vi "Text control 2 v0.3.vi"() -> ()   [LabVIEW 2016]
panel:
  out "Ion vs time":cluster{"Y data in":dbl[], "X data in":dbl[]}[](graph)
  out "Ig":dbl format="%.2e"
  out "Id":dbl format="%.2e"
  out "Is":dbl format="%.2e"
  out "I vs Vg":cluster{"Y data in":dbl[], "X data in":dbl[]}[](graph)
  in  "Suffix":string=".txt"
  in  "Prefix":string="-transfer-"
  in  "Panel Controls 2":T1={"Emergency Stop"=refnum, "TransGraph Max"=1e-05, "Text/Graph (text=false)"=TRUE, "TransGraph Min"=1e-11} {"TransGraph Min" format="%.2e"; "TransGraph Max" format="%.2e"}
  out "Currently running:":string="#output s 0 0 0 -0.008 0.008 0.002"
  in  "Lines left to run:":string
  in  "Standby":T2
  in  "Full Reset":bool
  in  "SMU4":cluster{"on/off":bool, "Voltage":dbl} {"Voltage" min=-100.0 max=100.0 format="%.2f"}
  in  "Source/Drain\nRange":u8(slide)=6 max=11 scale=0.0..11.0
  in  "Source/Drain\nRange mode":u16(ring) items=["Auto", "Limited", "Fixed"]
  in  "Gate Range":u8(slide)=6 max=11 scale=0.0..11.0
  in  "Gate Range\nmode":u16(ring) items=["Auto", "Limited", "Fixed"]
  in  "Gate":T3={"Gate Start"=0.0, "Gate Stop"=2.0, "Gate Step (linear only)"=1.0, "Gate Compliance"=0.0001, "Gate PComp"=0.0, "Range mode"=0, "Range"=6} {"Range" max=11 scale=0.0..11.0; "Range mode" items=["Auto", "Limited", "Fixed"]; "Gate PComp" format="%^.2e"; "Gate Compliance" format="%^.2e"; "Gate Step (linear only)" format="%^.4e"; "Gate Stop" format="%^.4e"; "Gate Start" format="%^.4e"}
  in  "Drain 2":T4={"Drain Start"=0.0, "Drain Stop"=2.0, "Drain Compliance"=0.0001, "Drain Step"=1.0, "Drain PComp"=0.0, "Range mode"=0, "Range"=6} {"Range" max=11 scale=0.0..11.0; "Range mode" items=["Auto", "Limited", "Fixed"]; "Drain PComp" format="%^.2e"; "Drain Step" format="%^.4e"; "Drain Compliance" format="%^.2e"; "Drain Stop" format="%^.4e"; "Drain Start" format="%^.4e"}
  in  "Timings 2":T5={"integration time"=0, "Short/Long integration time"=0.00064, "hold time (sec)"=0.0, "delay time (sec)"=0.0, "Step Time (0 disables)"=0.0, "sweep method"=0, "Pulse period"=0.005, "Base voltage"=0.0, "Pulse width"=0.0005} {"Pulse width" min=0.0005 max=0.1 step=0.0001 format="%.4f"; "Base voltage" format="%^.4e"; "Pulse period" min=0.005 max=1.0 step=0.0001 format="%.4f"; "sweep method" items=["Continuous", "Pulsed"]; "Step Time (0 disables)" format="%.2f"; "delay time (sec)" format="%.4f"; "hold time (sec)" format="%.4f"; "Short/Long integration time" format="%^.0e"; "integration time" scale=0.0..2.0}
  in  "Panel Controls":T6={"Emergency Stop"=refnum, "TransGraph Max"=1e-05, "Text/Graph (text=false)"=TRUE} {"TransGraph Max" format="%.2e"}
  in  "Interrupt run":bool
  in  "Drain: Compliance":dbl=0.001 format="%.8f"
  in  "Gate: Compliance":dbl=0.001 format="%.8f"
  out "Path":path=path "C:/users/rlp38/09Apr2009LTtesting/test2.txt"
  in  "hold time /s":dbl format="%.2f"
  in  "delay time /s":dbl format="%.2f"
  in  "integration time":u32(slide) max=2 step=1 scale=0.0..2.0
  in  "Integration time (short)":dbl=0.0019 min=8e-05 max=0.0019 step=8e-05 format="%^.0e"
  in  "Integration time (long)":dbl=0.32 min=0.04 max=2.0 step=0.02 format="%.2f"
  in  "Step delay /s":dbl format="%.2f"
  in  "Program":string="#pulsedstressV d 0.03 20 0 0.5 0.0827 5\n#\n#itime m\n#gaterangemode a\n#drainrangemode a\n#pulsed on 0.05 0 0.02\n#transfer d -10 40 1 5 40 35\n#transfer d -10 40 1 5 40 35\n#transfer d -10 40 1 5 40 35\n#output d 0 40 20 0 40 1\n#\n#\n#sample 1 0.008 221 6 0.003\n#samplei 400e-6 200 6 0.002 0.1\n#vsu2pulse -10 4\n#\n#stressV 0.016 0.03 2e-4 0.1e-3 11\n#stressI 220e-7 0.08 15\n#transfer s -1 1 0.5 -0.005 0.005 0.005\n#output s 0 0 0 -0.008 0.008 0.002\n"
  # "Syntax:\nitime [s|m|l]\ngaterangemode [a|l|f]\ndrainrangemode [a|l|f]\npulsed [on|off] PulsePeriod(sec) PulseBaseVoltage PulseONWidth(sec)\nstandby [on l off]\nwait NumMilliseconds\nwait-min NumMinutes\n# texthere = comment\ntransfer [s|d] VgStart VgStop VgStep VdStart VdStop VdStep\noutput [s|d] VgStart VgStop VgStep VdStart VdStop VdStep\nsample Vg Vd NumSamples Time(s) SampleInterval(s)\nsamplei Idg NumSamples Time(s) SampleInterval(s) VDGcompliance\n# if in doubt use SampleInterval(s) = 0.004\nstressV VG VD IGcompliance IDcompliance Duration(sec)\nstressI IDG VDGcompliance Duration(sec)\nvsu2pulse Bias Duration(s)\npulsedstressV [s|d] VEstop VgON VgOFF Period(s) PulseONwidth(s) Vd\nsample-fpp Vg Vd NumSamples Time\nresample-fpp Vg Vd\ntransfer-fpp [s|d] VgStart VgStop VgStep VdStart VdStop VdStep\noutput-fpp [s|d] VgStart VgStop VgStep VdStart VdStop VdStep"
  # "100 samples is approx 13s with medium integration"
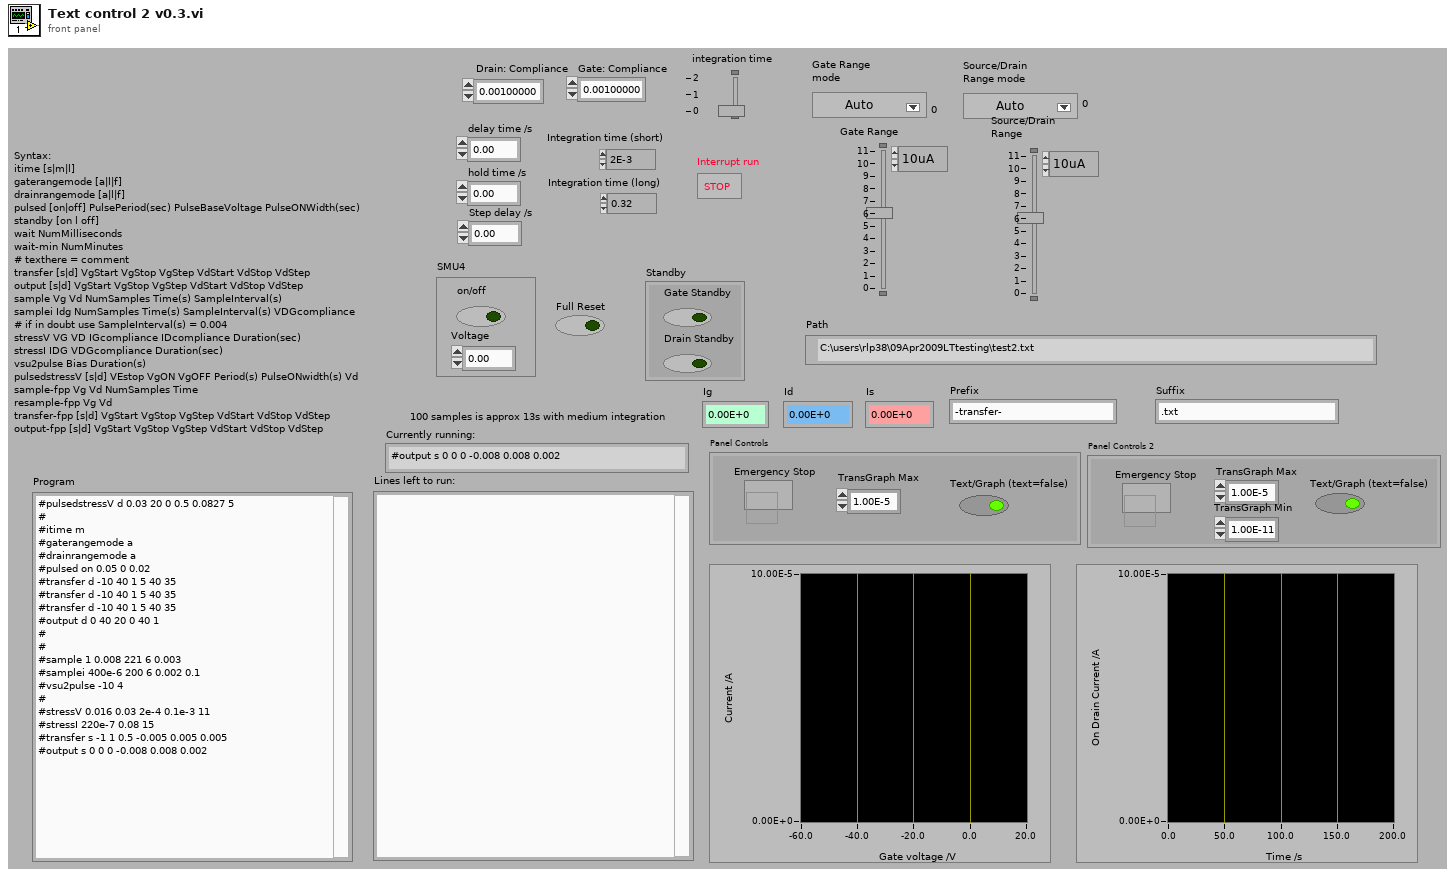
[diagram p1: front panel]
types:
  T1 = cluster{"Emergency Stop":refnum<vi>, "TransGraph Max":dbl, "Text/Graph (text=false)":bool, "TransGraph Min":dbl}
  T2 = cluster{"Gate Standby":bool, "Drain Standby":bool}
  T3 = cluster{"Gate Start":dbl, "Gate Stop":dbl, "Gate Step (linear only)":dbl, "Gate Compliance":dbl, "Gate PComp":dbl, "Range mode":u16, "Range":u8}
  T4 = cluster{"Drain Start":dbl, "Drain Stop":dbl, "Drain Compliance":dbl, "Drain Step":dbl, "Drain PComp":dbl, "Range mode":u16, "Range":u8}
  T5 = cluster{"integration time":u32, "Short/Long integration time":dbl, "hold time (sec)":dbl, "delay time (sec)":dbl, "Step Time (0 disables)":dbl, "sweep method":u16, "Pulse period":dbl, "Base voltage":dbl, "Pulse width":dbl}
  T6 = cluster{"Emergency Stop":refnum<vi>, "TransGraph Max":dbl, "Text/Graph (text=false)":bool}
  T7 = enum16{"open", "replace", "create", "open or create", "replace or create", "replace or create with confirmation"}
  T8 = cluster{"V2 Start":dbl, "V2 Step":dbl, "Number of points":i32}
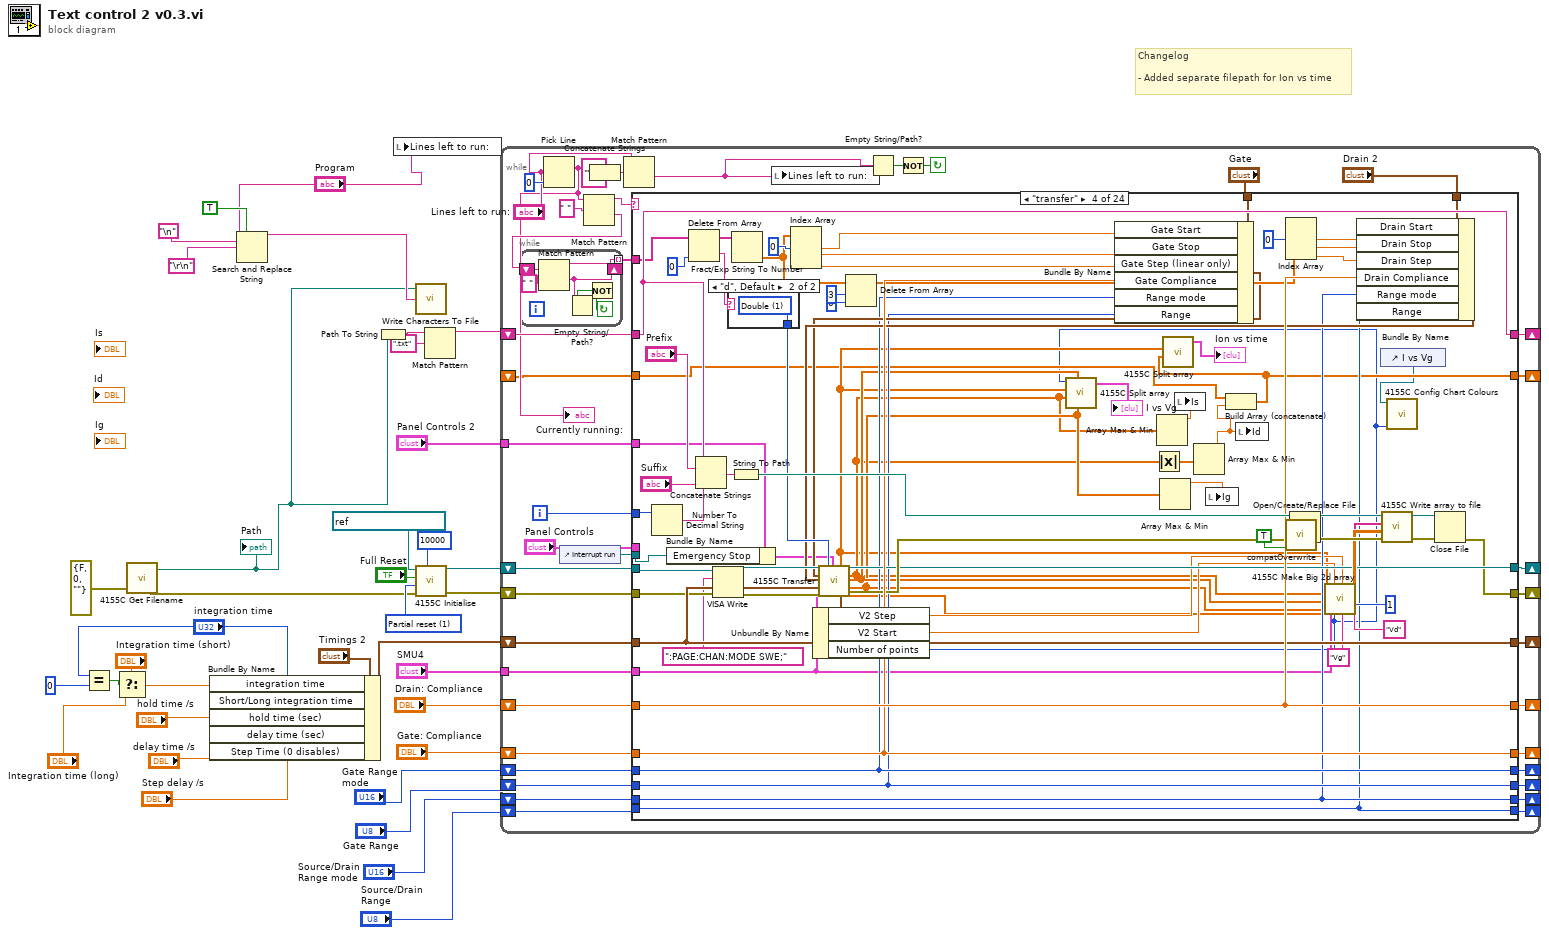
[diagram p0: block diagram]
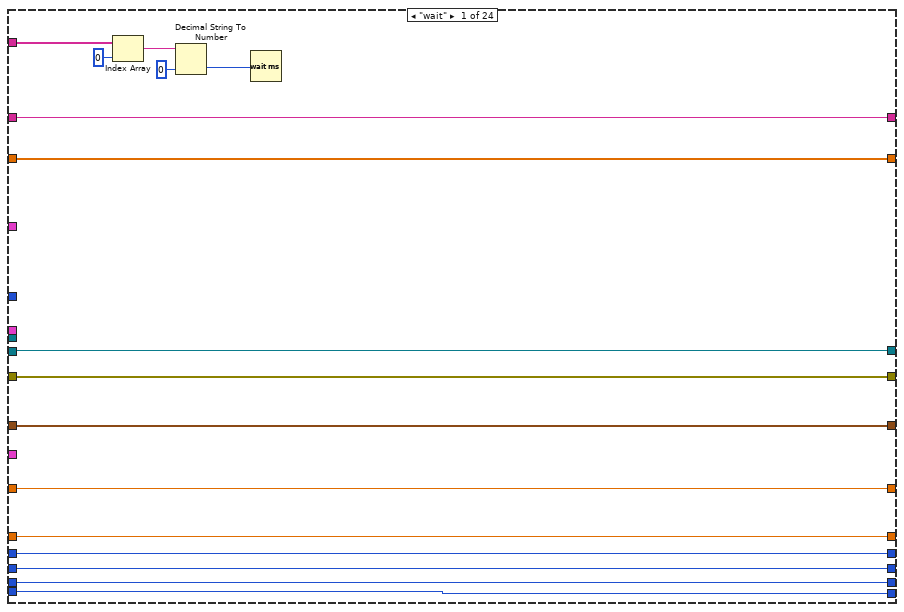
[diagram p2: hidden frame]
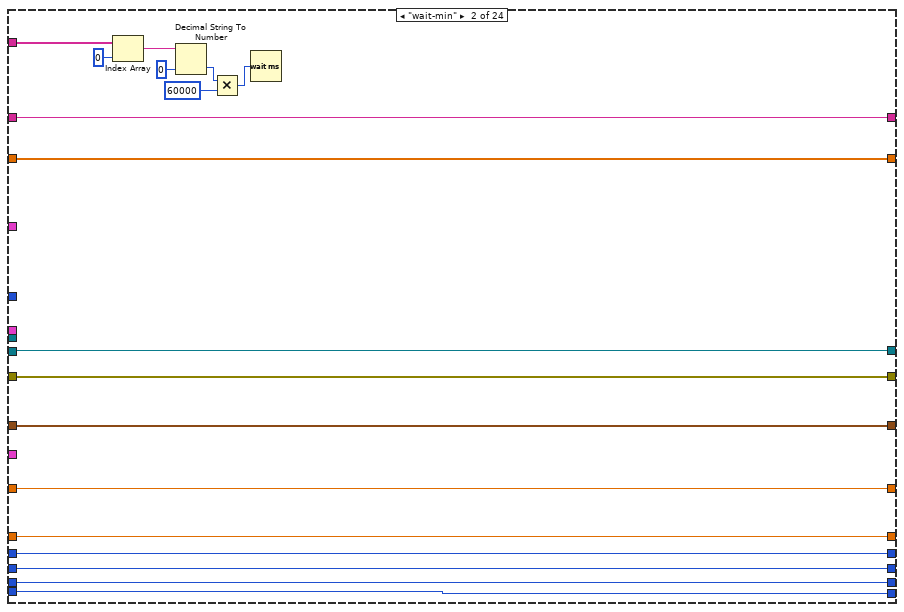
[diagram p3: hidden frame]
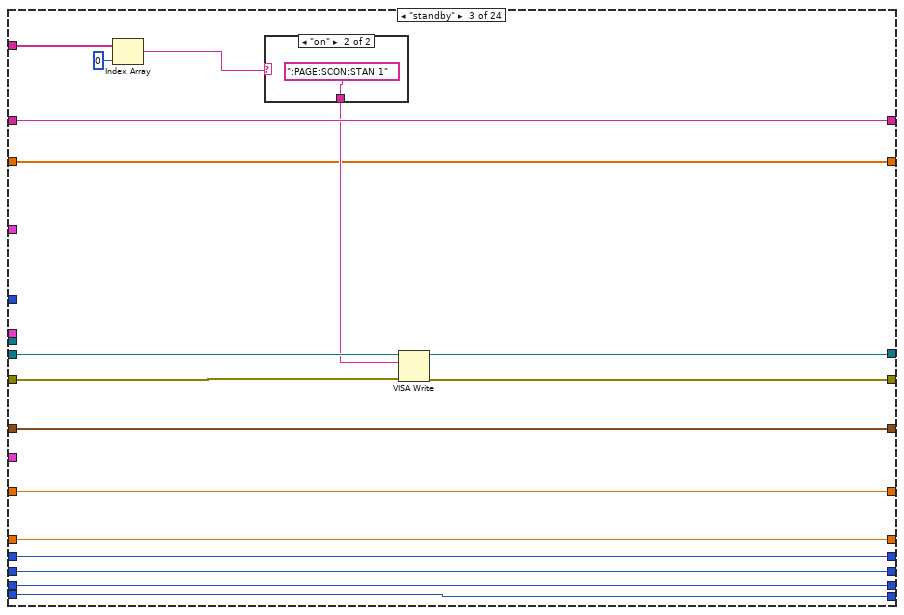
[diagram p4: hidden frame]
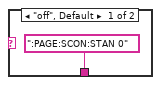
[diagram p5: hidden frame]
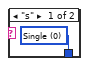
[diagram p6: hidden frame]
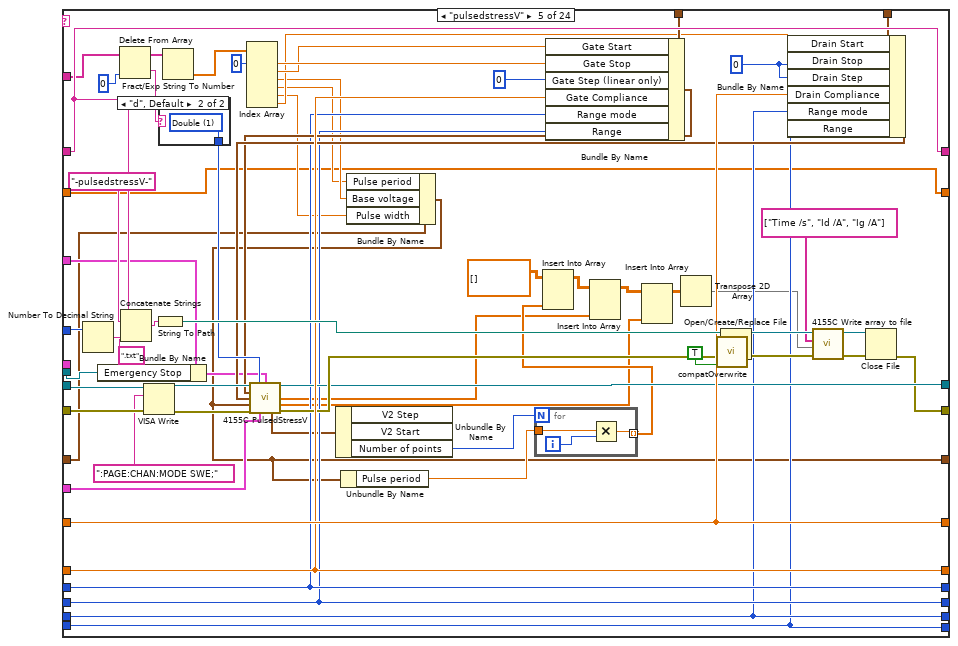
[diagram p7: hidden frame]
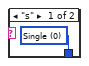
[diagram p8: hidden frame]
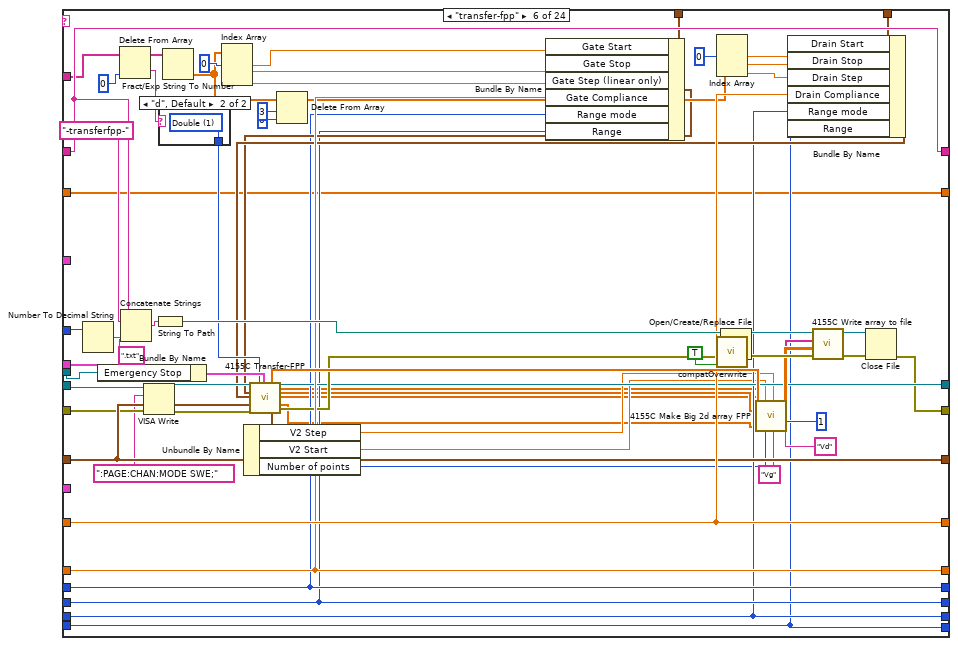
[diagram p9: hidden frame]
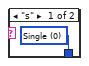
[diagram p10: hidden frame]
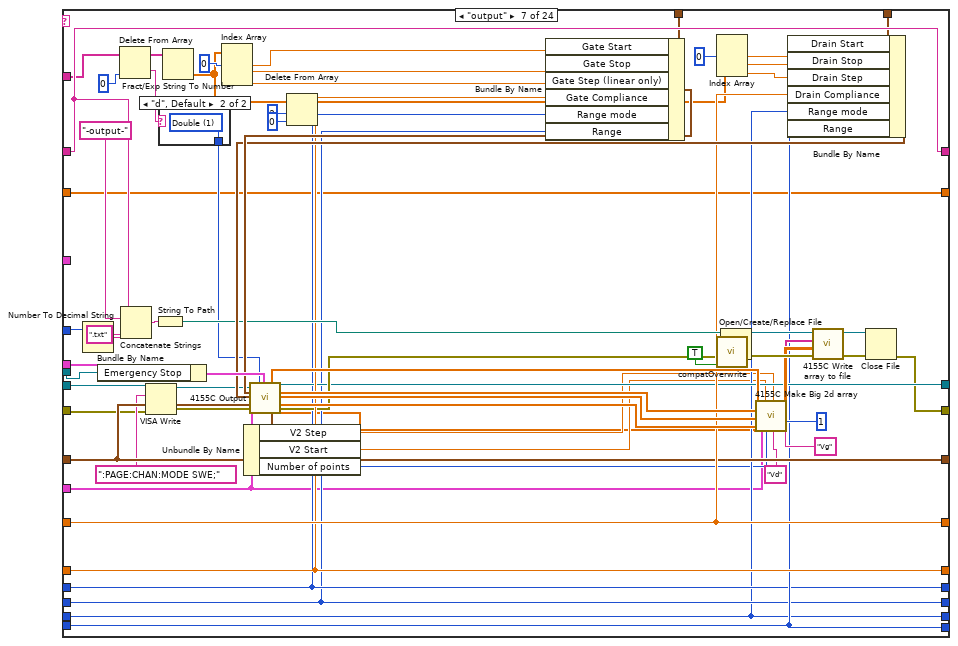
[diagram p11: hidden frame]
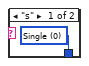
[diagram p12: hidden frame]
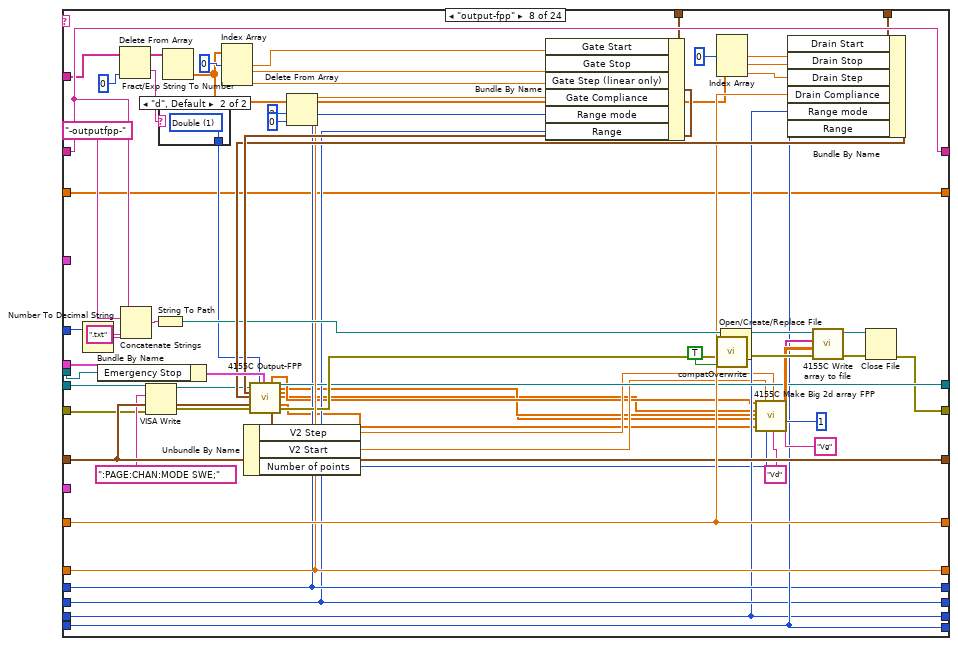
[diagram p13: hidden frame]
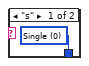
[diagram p14: hidden frame]
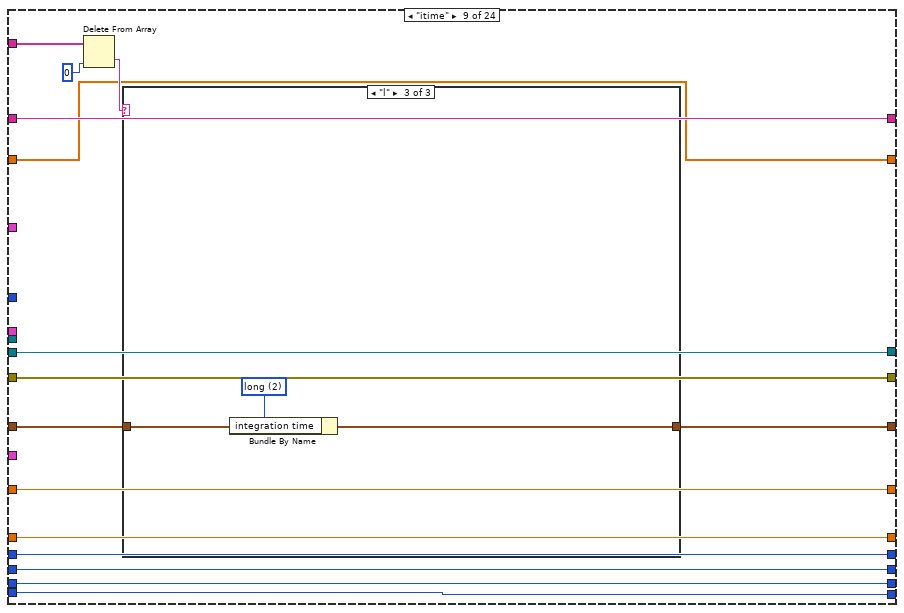
[diagram p15: hidden frame]
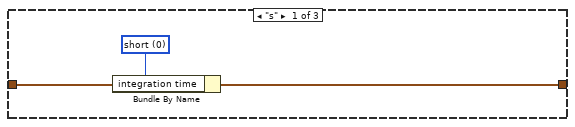
[diagram p16: hidden frame]
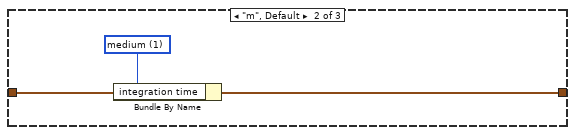
[diagram p17: hidden frame]
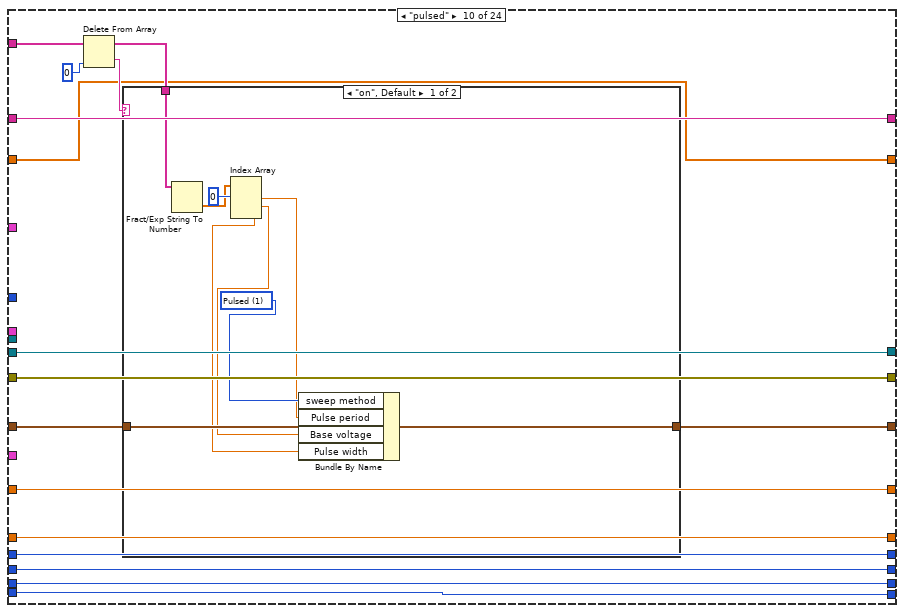
[diagram p18: hidden frame]
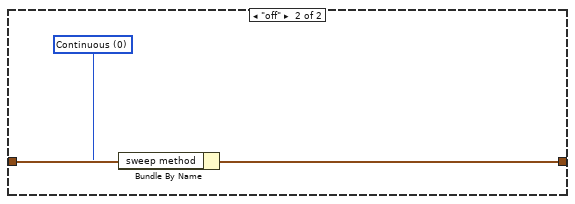
[diagram p19: hidden frame]
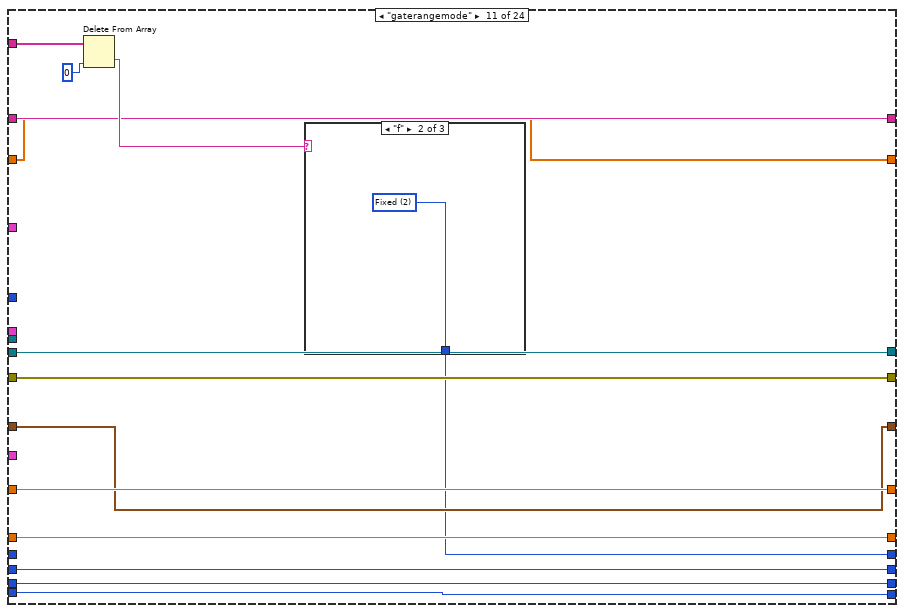
[diagram p20: hidden frame]
diagram:
  w27 = u16 1 items=["Reset All", "Partial reset"] ("Type of reset")
  # "Changelog\n\n- Added separate filepath for Ion vs time"
  n1 = Equal?(x="integration time", y=u32 0) -> (x = y?=w31:bool)
  n2 = Select(t="Integration time (short)", s=w31, f="Integration time (long)") -> (s? t:f=w35:dbl)
  n3 = call <userlib>:"4155C Get Filename.vi"("error in (no error)"=errorcluster {"status"=FALSE, "code"=0, "source"=""}) -> ("error out"=w22:errorcluster, "path"=w6:path)  [unwired: 2 in, 1 out]
  "Path" <- w6
  n4 = Bundle By Name(cluster="Timings 2", "integration time"="integration time", "Short/Long integration time"=w35, "hold time (sec)"="hold time /s", "delay time (sec)"="delay time /s", "Step Time (0 disables)"="Step delay /s") -> (w19:T5)
  n5 = Search and Replace String(replace all?=TRUE ("replace all? (F)"), input string="Program", search string="\n", replace string="\r\n") -> (result string=w9:string)  [unwired: 4 in, 3 out]
  n6 = Path To String(path=w6) -> (string=w5:string)
  n7 = local write "Lines left to run:"("Program") -> ()
  n8 = call <vilib>:"Write Characters To File.vi"("character string"=w9, "file path (dialog if empty)"=w6) -> ()  [unwired: 3 in, 1 out]
  n9 = call <userlib>:"4155C Initialise.vi"("VISA resource name in"=refnum<visa-resource-name> "GPIB0::14::INSTR", "Reset"="Full Reset", "Type of reset"=w27, "error in (no error)"=w22, "VISA Timeout Value"=u32 10000) -> ("VISA Resource Name out"=w21:refnum<visa-resource-name>, "error out"=w20:errorcluster)
  n10 = Match Pattern(string=w5, regular expression=".txt") -> (before substring=w4:string)  [unwired: 1 in, 3 out]
  n11 = while {
    tunnel: "SMU4" -> [w43]
    shift-left: "Source/Drain\nRange" -> [w48]
    shift-right: [w44] -> _
    shift-left: "Source/Drain\nRange mode" -> [w49]
    shift-right: [w45] -> _
    shift-left: "Gate Range" -> [w50]
    shift-right: [w46] -> _
    shift-left: "Gate Range\nmode" -> [w51]
    shift-right: [w47] -> _
    shift-left: "Gate: Compliance" -> [w63]
    shift-right: [w57] -> _
    shift-left: "Drain: Compliance" -> [w64]
    shift-right: [w58] -> _
    shift-left: w19 -> [w65]
    shift-right: [w59] -> _
    shift-left: w20 -> [w66]
    shift-right: [w60] -> _
    shift-left: w21 -> [w67]
    shift-right: [w61] -> _
    shift-left: w4 -> [w68]
    shift-right: [w56] -> _
    tunnel: "Panel Controls 2" -> [w39]
    shift-right: [w38] -> _
    shift-left: _ -> [w37]
    i -> [w62]
    stop <- w76 continue-if-true
    n12 = Pick Line(multi-line string="Lines left to run:", line index=0) -> (output string=w40:string)  [unwired: 1 in]
    "Currently running:" <- w40
    n13 = control-ref of="Interrupt run"() -> (w55:refnum<vi>)
    n14 = Match Pattern(string=w40, regular expression=" ") -> (before substring=w71:string, after substring=w70:string)  [unwired: 1 in, 2 out]
    n15 = while {
      tunnel: [w78] -> w69 mode=indexing
      shift-left: w70 -> [w80]
      shift-right: [w79] -> _
      stop <- w82 continue-if-true
      n16 = Match Pattern(string=w80, regular expression=" ") -> (before substring=w78:string, after substring=w79:string)  [unwired: 1 in, 2 out]
      n17 = Empty String/Path?(string/path=w79) -> (empty?=w83:bool)
      n18 = Not(x=w83) -> (.not. x?=w82:bool)
    }
    n19 = Concatenate Strings(w40, "\n" ("Substring")) -> (w74:string)
    n20 = Match Pattern(string="Lines left to run:", regular expression=w74) -> (after substring=w41:string)  [unwired: 1 in, 3 out]
    n21 = case shown="\"transfer\"" w71 {
      tunnel: w69 -> [w99 w117 w134 w193 w262 w329 w394 w467 w505 w530 w556 w580 w600 w613 _ _ w711 w770 _ w832 w874 w914 w982 w1042]
      tunnel: w68 -> [w94 w113 w132 w201 w269 w337 w402 w475 w494 w519 w548 w573 w594 w606 w624 w663 w689 w752 w783 w819 w861 w902 w976 w1038]
      tunnel: w67 -> [w93 w112 w123 w171 w253 w306 w370 w443 w495 w520 w549 w574 w595 w607 w629 w666 w718 w777 w787 w839 w881 w921 w989 w995]
      tunnel: w66 -> [w92 w111 w122 w170 w252 w305 w367 w440 w496 w521 w550 w575 w596 w608 w628 w635 w717 w776 w786 w838 w880 w920 w988 w994]
      tunnel: w65 -> [w91 w110 w131 w197 w227 w333 w398 w471 w504 w529 w547 w572 w593 w605 w627 w659 w680 w744 w792 w812 w854 w895 w975 w1037]
      tunnel: w64 -> [w90 w109 w130 w199 w267 w335 w400 w473 w503 w528 w555 w579 w599 w612 w626 w644 w716 w775 w795 w837 w879 w919 w987 w1047]
      tunnel: w63 -> [w89 w108 w129 w198 w266 w334 w399 w472 w502 w527 w554 w578 w598 w611 w625 w645 w690 w753 w794 w820 w862 w903 w977 w1039]
      tunnel: w62 -> [_ _ _ w139 w270 w338 w403 w476 _ _ _ _ _ _ _ w661 w715 w774 _ w836 w878 w918 w986 w1046]
      tunnel: [w93 w112 w121 w195 w264 w331 w396 w469 w495 w520 w549 w574 w595 w607 w629 w666 w681 w725 w785 w813 w855 w896 w927 w997] -> w61
      tunnel: [w92 w111 w120 w194 w263 w330 w395 w468 w496 w521 w550 w575 w596 w608 w628 w634 w691 w726 w784 w821 w863 w904 w926 w996] -> w60
      tunnel: [w91 w110 w131 w197 w223 w333 w398 w471 w497 w522 w547 w572 w593 w605 w627 w659 w680 w744 w792 w812 w854 w895 w975 w1037] -> w59
      tunnel: [w90 w109 w130 w199 w267 w335 w400 w473 w503 w528 w555 w579 w599 w612 w626 w644 w716 w775 w795 w837 w879 w919 w987 w1047] -> w58
      tunnel: [w89 w108 w129 w198 w266 w334 w399 w472 w502 w527 w554 w578 w598 w611 w625 w645 w690 w753 w794 w820 w862 w903 w977 w1039] -> w57
      tunnel: [w94 w113 w132 w201 w269 w337 w402 w475 w494 w519 w548 w573 w594 w606 w624 w663 w689 w752 w783 w819 w861 w902 w976 w1038] -> w56
      tunnel: w55 -> [_ _ _ w205 w274 w343 w411 w480 _ _ _ _ _ _ _ _ w686 w749 _ w818 w860 w901 w947 w1013]
      tunnel: "Gate" -> [_ _ _ w180 w256 w316 w381 w454 _ _ _ _ _ _ _ _ _ _ _ _ _ _ _ _]
      tunnel: "Drain 2" -> [_ _ _ w179 w255 w315 w380 w453 _ _ _ _ _ _ _ _ _ _ _ _ _ _ _ _]
      tunnel: "Panel Controls" -> [_ _ _ _ _ w314 w379 w452 _ _ _ _ _ _ _ _ _ _ _ _ _ _ _ _]
      tunnel: w51 -> [w88 w107 w128 w164 w246 w299 w365 w438 w501 w526 _ w571 w592 w604 w623 w646 w676 w740 w788 w808 w850 w891 w971 w1033]
      tunnel: w50 -> [w87 w106 w127 w163 w245 w298 w364 w437 w500 w525 w553 _ w583 w610 w622 w647 w677 w741 w789 w809 w851 w892 w972 w1034]
      tunnel: w49 -> [w86 w105 w126 w162 w244 w297 w363 w436 w499 w524 w552 w577 w597 _ w621 w648 w678 w742 w790 w810 w852 w893 w973 w1035]
      tunnel: w48 -> [w85 w104 w125 w161 w243 w296 w366 w439 w498 w523 w551 w576 _ w609 w620 w649 w679 w743 w791 w811 w853 w894 w974 w1036]
      tunnel: [w88 w107 w128 w164 w246 w299 w365 w438 w501 w526 w546 w571 w592 w604 w623 w646 w676 w740 w788 w808 w850 w891 w971 w1033] -> w47
      tunnel: [w87 w106 w127 w163 w245 w298 w364 w437 w500 w525 w553 w563 w583 w610 w622 w647 w677 w741 w789 w809 w851 w892 w972 w1034] -> w46
      tunnel: [w86 w105 w126 w162 w244 w297 w363 w436 w499 w524 w552 w577 w597 w603 w621 w648 w678 w742 w790 w810 w852 w893 w973 w1035] -> w45
      tunnel: [w85 w104 w125 w161 w243 w296 w366 w439 w498 w523 w551 w576 w584 w609 w620 w649 w679 w743 w791 w811 w853 w894 w974 w1036] -> w44
      tunnel: w43 -> [_ _ _ w155 w239 _ w357 _ _ _ _ _ _ _ _ _ _ _ _ _ _ _ _ _]
      tunnel: w39 -> [_ _ _ w153 w238 _ _ _ _ _ _ _ _ _ _ _ _ _ _ _ _ _ _ _]
      tunnel: [w84 w100 w118 w142 w215 w285 w354 w424 w493 w517 w545 w562 w582 w602 w619 w630 w667 w723 w782 w796 w842 w884 w924 w990] -> w38
      tunnel: w37 -> [w84 w100 w118 w141 w215 w285 w354 w424 w493 w517 w545 w562 w582 w602 w619 w630 w667 w723 w782 w796 w842 w884 w924 w990]
      frame "wait" {
        n22 = Index Array(array=w99, index=0 ("Index")) -> (element=w97:string)
        n23 = Decimal String To Number(string=w97, default (0L)=u32 0) -> (number=w96:u32)  [unwired: 1 in, 1 out]
        n24 = Wait (ms)(milliseconds to wait=w96) -> ()  [unwired: 1 out]
      }
      frame "wait-min" {
        n25 = Index Array(array=w117, index=0 ("Index")) -> (element=w115:string)
        n26 = Decimal String To Number(string=w115, default (0L)=u32 0) -> (number=w103:u32)  [unwired: 1 in, 1 out]
        n27 = Multiply(x=w103, y=u32 60000) -> (x*y=w102:u32)
        n28 = Wait (ms)(milliseconds to wait=w102) -> ()  [unwired: 1 out]
      }
      frame "standby" {
        n29 = Index Array(array=w134, index=0 ("Index")) -> (element=w124:string)
        n30 = case shown="\"on\"" w124 {
          tunnel: [":PAGE:SCON:STAN 0" ":PAGE:SCON:STAN 1"] -> w119
          frame "off", Default {
          }
          frame "on" {
          }
        }
        n31 = VISA Write(VISA resource name=w123, write buffer=w119, error in (no error)=w122) -> (VISA resource name out=w121:refnum<visa-resource-name>, error out=w120:errorcluster)  [unwired: 1 out]
      }
      frame "transfer" {
        n32 = Number To Decimal String(number=w139) -> (decimal integer string=w202:string)  [unwired: 1 in]
        n33 = Bundle By Name(cluster=w153, "Emergency Stop"=w205) -> (w154:T1)
        n34 = Delete From Array(array=w193, index=0 ("Index")) -> (deleted portion=w191:string, array with subset deleted=w190:string[])  [unwired: 1 in]
        n35 = Concatenate Strings(w201, "Prefix", w202, "Suffix") -> (w204:string)
        n36 = VISA Write(VISA resource name=w171, write buffer=":PAGE:CHAN:MODE SWE;" ("write buffer (\"\")"), error in (no error)=w170) -> (VISA resource name out=w168:refnum<visa-resource-name>, error out=w169:errorcluster)  [unwired: 1 out]
        n37 = case shown="\"d\", Default" w191 {
          tunnel: [w213 w214] -> w189
          frame "s" {
            w213 = u16 0 items=["Single", "Double"] ("sweep mode")
          }
          frame "d", Default {
            w214 = u16 1 items=["Single", "Double"] ("sweep mode")
          }
        }
        n38 = String To Path(string=w204) -> (path=w200:path)
        n39 = Fract/Exp String To Number(string=w190) -> (number=w175:dbl[])  [unwired: 3 in, 1 out]
        n40 = Index Array(array=w175, index #1=0 ("Index")) -> (element #1=w188:dbl, element #2=w187:dbl, element #3=w186:dbl)  [unwired: 2 in]
        n41 = Delete From Array(array=w175, length=3 ("Length"), index=0 ("Index")) -> (array with subset deleted=w173:dbl[])  [unwired: 1 out]
        n42 = Bundle By Name(cluster=w180, "Gate Start"=w188, "Gate Stop"=w187, "Gate Step (linear only)"=w186, "Gate Compliance"=w198, "Range mode"=w164, "Range"=w163) -> (w165:T3)
        n43 = Index Array(array=w173, index #1=0 ("Index")) -> (element #1=w183:dbl, element #2=w182:dbl, element #3=w181:dbl)  [unwired: 2 in]
        n44 = call <vilib>:"compatOverwrite.vi"("overwrite (F)"=TRUE) -> ("overwrite?"=w152:T7)
        n45 = Bundle By Name(cluster=w179, "Drain Start"=w183, "Drain Stop"=w182, "Drain Step"=w181, "Drain Compliance"=w199, "Range mode"=w162, "Range"=w161) -> (w166:T4)
        n46 = call <userlib>:"4155C Transfer.vi"("VISA resource name in"=w168, "Gate"=w165, "Drain"=w166, "Timings"=w197, "error in (no error)"=w169, "SMU4"=w155, "sweep mode"=w189, "Panel Controls"=w154) -> ("VG"=w143:dbl[], "Outparams"=w159:T8, "VISA Resource Name out"=w195:refnum<visa-resource-name>, "IS"=w145:dbl[], "ID"=w150:dbl[], "IG"=w146:dbl[], "error out"=w196:errorcluster, "SMU4"=w156:dbl[])  [unwired: 12 in]
        n47 = Unbundle By Name(w159) -> ("V2 Step"=w158:dbl, "V2 Start"=w157:dbl, "Number of points"=w138:i32)
        n48 = call <userlib>:"4155C Split array.vi"("Number of VAR2 steps"=w138, "Y2 data in"=w150, "X data in"=w143, "Y1 data in"=w145, "Y3 data in"=w146) -> ("Array of clusters"=→"I vs Vg":cluster{"Y data in":dbl[], "X data in":dbl[]}[])  [unwired: 2 in, 1 out]
        n49 = Absolute Value(x=w145) -> (abs(x)=w149:dbl[])
        n50 = Array Max & Min(array=w145) -> (max value=w147:dbl)  [unwired: 3 out]
        n51 = Array Max & Min(array=w146) -> (max value=w148:dbl)  [unwired: 3 out]
        n52 = local write "Is"(w147) -> ()
        n53 = Array Max & Min(array=w149) -> (max value=w140:dbl)  [unwired: 3 out]
        n54 = local write "Ig"(w148) -> ()
        n55 = Build Array (concatenate)(w141, w140) -> (w142:dbl[])
        n56 = call <userlib>:"4155C Split array.vi"("X data in"=w143, "Y1 data in"=w142) -> ("Array of clusters"=→"Ion vs time":cluster{"Y data in":dbl[], "X data in":dbl[]}[])  [unwired: 5 in, 1 out]
        n57 = local write "Id"(w140) -> ()
        n58 = Open/Create/Replace File(file path (use dialog)=w200, error in=w196, operation (0:open)=w152) -> (refnum out=w210:refnum<file>, error out=w211:errorcluster)  [unwired: 3 in, 1 out]
        n59 = call <userlib>:"4155C Make Big 2d array.vi"("1D Var1"=w143, "1d IS"=w145, "1d ID"=w150, "1d IG"=w146, "1d SMU4"=w156, "SMU4"=w155, "VAR2 START"=w157, "Number of VAR2 steps"=w138, "VAR2 STEP"=w158, "VAR1 Name"="Vg", "Decimal places in header"=i8 1, "VAR2 Name"="Vd") -> ("Header array"=w206:string[], "Data array"=w207:dbl[][])  [unwired: 14 in]
        n60 = control-ref of="I vs Vg"() -> (w137:refnum<vi>)
        n61 = call <userlib>:"4155C Write array to file.vi"("Byte Stream File Refnum"=w210, "Header"=w206, "Data Array"=w207, "error in (no error)"=w211) -> ("dup refnum"=w208:refnum<file>, "error out"=w209:errorcluster)  [unwired: 1 in]
        n62 = call <userlib>:"4155C Config Chart Colours.vi"("Numeric"=w138, "XY Graph 2"=w137) -> ()  [unwired: 6 in]
        n63 = Close File(refnum=w208, error in=w209) -> (error out=w194:errorcluster)  [unwired: 1 out]
      }
      frame "pulsedstressV" {
        w221 = 0
        n64 = Number To Decimal String(number=w270) -> (decimal integer string=w271:string)  [unwired: 1 in]
        n65 = Bundle By Name(cluster=w238, "Emergency Stop"=w274) -> (w240:T1)
        n66 = Delete From Array(array=w262, index=0 ("Index")) -> (deleted portion=w260:string, array with subset deleted=w259:string[])  [unwired: 1 in]
        n67 = Concatenate Strings(w269, "-pulsedstressV-" ("Substring"), w271, ".txt" ("Substring")) -> (w273:string)
        n68 = VISA Write(VISA resource name=w253, write buffer=":PAGE:CHAN:MODE SWE;" ("write buffer (\"\")"), error in (no error)=w252) -> (VISA resource name out=w250:refnum<visa-resource-name>, error out=w251:errorcluster)  [unwired: 1 out]
        n69 = String To Path(string=w273) -> (path=w268:path)
        n70 = case shown="\"d\", Default" w260 {
          tunnel: [w283 w284] -> w258
          frame "s" {
            w283 = u16 0 items=["Single", "Double"] ("sweep mode")
          }
          frame "d", Default {
            w284 = u16 1 items=["Single", "Double"] ("sweep mode")
          }
        }
        n71 = Fract/Exp String To Number(string=w259) -> (number=w254:dbl[])  [unwired: 3 in, 1 out]
        n72 = Index Array(array=w254, index #1=0 ("Index")) -> (element #1=w230:dbl, element #2=w229:dbl, element #3=w226:dbl, element #4=w225:dbl, element #5=w224:dbl, element #6=w228:dbl)  [unwired: 5 in]
        n73 = Bundle By Name(cluster=w227, "Pulse period"=w225, "Base voltage"=w226, "Pulse width"=w224) -> (w223:T5)
        n74 = Unbundle By Name(w223) -> ("Pulse period"=w231:dbl)
        n75 = Bundle By Name(cluster=w256, "Gate Start"=w229, "Gate Stop"=w230, "Gate Step (linear only)"=0, "Gate Compliance"=w266, "Range mode"=w246, "Range"=w245) -> (w247:T3)
        n76 = call <vilib>:"compatOverwrite.vi"("overwrite (F)"=TRUE) -> ("overwrite?"=w216:T7)
        n77 = Bundle By Name(cluster=w255, "Drain Start"=w228, "Drain Stop"=w221, "Drain Step"=w221, "Drain Compliance"=w267, "Range mode"=w244, "Range"=w243) -> (w248:T4)
        n78 = call <userlib>:"4155C PulsedStressV.vi"("VISA resource name in"=w250, "sweep mode"=w258, "Panel Controls"=w240, "Gate"=w247, "Drain"=w248, "Timings"=w223, "error in (no error)"=w251, "SMU4"=w239) -> ("VISA Resource Name out"=w264:refnum<visa-resource-name>, "ID"=w219:dbl[], "IG"=w217:dbl[], "Outparams"=w241:T8, "error out"=w265:errorcluster)  [unwired: 3 in]
        n79 = Unbundle By Name(w241) -> ("Number of points"=w218:i32)  [unwired: 2 out]
        n80 = for {
          N: w218 -> [_]
          tunnel: [w280] -> w220 mode=indexing
          tunnel: w231 -> [w282]
          i -> [w281]
          n81 = Multiply(x=w282, y=w281) -> (x*y=w280:dbl)
        }
        n82 = Insert Into Array(array=dbl[][] [] ("Input Array"), new element=w220) -> (w232:dbl[][])  [unwired: 2 in]
        n83 = Insert Into Array(array=w232, new element=w219) -> (w237:dbl[][])  [unwired: 2 in]
        n84 = Insert Into Array(array=w237, new element=w217) -> (w236:dbl[][])  [unwired: 2 in]
        n85 = Transpose 2D Array(2D array=w236) -> (transposed array=w235:dbl[][])
        n86 = Open/Create/Replace File(file path (use dialog)=w268, error in=w265, operation (0:open)=w216) -> (refnum out=w277:refnum<file>, error out=w278:errorcluster)  [unwired: 3 in, 1 out]
        n87 = call <userlib>:"4155C Write array to file.vi"("Byte Stream File Refnum"=w277, "Header"=string[] ["Time /s", "Id /A", "Ig /A"], "Data Array"=w235, "error in (no error)"=w278) -> ("dup refnum"=w275:refnum<file>, "error out"=w276:errorcluster)  [unwired: 1 in]
        n88 = Close File(refnum=w275, error in=w276) -> (error out=w263:errorcluster)  [unwired: 1 out]
      }
      frame "transfer-fpp" {
        n89 = Number To Decimal String(number=w338) -> (decimal integer string=w339:string)  [unwired: 1 in]
        n90 = Bundle By Name(cluster=w314, "Emergency Stop"=w343) -> (w351:T6)
        n91 = Delete From Array(array=w329, index=0 ("Index")) -> (deleted portion=w327:string, array with subset deleted=w326:string[])  [unwired: 1 in]
        n92 = Concatenate Strings(w337, "-transferfpp-" ("Substring"), w339, ".txt" ("Substring")) -> (w341:string)
        n93 = VISA Write(VISA resource name=w306, write buffer=":PAGE:CHAN:MODE SWE;" ("write buffer (\"\")"), error in (no error)=w305) -> (VISA resource name out=w303:refnum<visa-resource-name>, error out=w304:errorcluster)  [unwired: 1 out]
        n94 = String To Path(string=w341) -> (path=w336:path)
        n95 = case shown="\"d\", Default" w327 {
          tunnel: [w352 w353] -> w325
          frame "s" {
            w352 = u16 0 items=["Single", "Double"] ("sweep mode")
          }
          frame "d", Default {
            w353 = u16 1 items=["Single", "Double"] ("sweep mode")
          }
        }
        n96 = Fract/Exp String To Number(string=w326) -> (number=w310:dbl[])  [unwired: 3 in, 1 out]
        n97 = Index Array(array=w310, index #1=0 ("Index")) -> (element #1=w324:dbl, element #2=w323:dbl, element #3=w322:dbl)  [unwired: 2 in]
        n98 = Delete From Array(array=w310, length=3 ("Length"), index=0 ("Index")) -> (array with subset deleted=w308:dbl[])  [unwired: 1 out]
        n99 = Bundle By Name(cluster=w316, "Gate Start"=w324, "Gate Stop"=w323, "Gate Step (linear only)"=w322, "Gate Compliance"=w334, "Range mode"=w299, "Range"=w298) -> (w300:T3)
        n100 = Index Array(array=w308, index #1=0 ("Index")) -> (element #1=w319:dbl, element #2=w318:dbl, element #3=w317:dbl)  [unwired: 2 in]
        n101 = call <vilib>:"compatOverwrite.vi"("overwrite (F)"=TRUE) -> ("overwrite?"=w286:T7)
        n102 = Bundle By Name(cluster=w315, "Drain Start"=w319, "Drain Stop"=w318, "Drain Step"=w317, "Drain Compliance"=w335, "Range mode"=w297, "Range"=w296) -> (w301:T4)
        n103 = call <userlib>:"4155C Transfer-FPP.vi"("VISA resource name in"=w303, "Gate"=w300, "Drain"=w301, "Timings"=w333, "error in (no error)"=w304, "sweep mode"=w325, "Panel Controls"=w351) -> ("VG"=w342:dbl[], "Outparams"=w294:T8, "VISA Resource Name out"=w331:refnum<visa-resource-name>, "Vprobe2"=w290:dbl[], "ID"=w289:dbl[], "IG"=w288:dbl[], "Vprobe1"=w287:dbl[], "error out"=w332:errorcluster)  [unwired: 13 in]
        n104 = Unbundle By Name(w294) -> ("V2 Step"=w293:dbl, "V2 Start"=w292:dbl, "Number of points"=w291:i32)
        n105 = Open/Create/Replace File(file path (use dialog)=w336, error in=w332, operation (0:open)=w286) -> (refnum out=w348:refnum<file>, error out=w349:errorcluster)  [unwired: 3 in, 1 out]
        n106 = call <userlib>:"4155C Make Big 2d array FPP.vi"("1D Var1"=w342, "1d ID"=w289, "1d Vp2"=w290, "1d IG"=w288, "1d Vp1"=w287, "VAR2 START"=w292, "Number of VAR2 steps"=w291, "VAR2 STEP"=w293, "VAR1 Name"="Vg", "Decimal places in header"=i8 1, "VAR2 Name"="Vd") -> ("Header array"=w344:string[], "Data array"=w345:dbl[][])  [unwired: 15 in]
        n107 = call <userlib>:"4155C Write array to file.vi"("Byte Stream File Refnum"=w348, "Header"=w344, "Data Array"=w345, "error in (no error)"=w349) -> ("dup refnum"=w346:refnum<file>, "error out"=w347:errorcluster)  [unwired: 1 in]
        n108 = Close File(refnum=w346, error in=w347) -> (error out=w330:errorcluster)  [unwired: 1 out]
      }
      frame "output" {
        n109 = Number To Decimal String(number=w403) -> (decimal integer string=w404:string)  [unwired: 1 in]
        n110 = Bundle By Name(cluster=w379, "Emergency Stop"=w411) -> (w421:T6)
        n111 = Delete From Array(array=w394, index=0 ("Index")) -> (deleted portion=w392:string, array with subset deleted=w391:string[])  [unwired: 1 in]
        n112 = Concatenate Strings(w402, "-output-" ("Substring"), w404, ".txt" ("Substring")) -> (w406:string)
        n113 = VISA Write(VISA resource name=w370, write buffer=":PAGE:CHAN:MODE SWE;" ("write buffer (\"\")"), error in (no error)=w367) -> (VISA resource name out=w369:refnum<visa-resource-name>, error out=w368:errorcluster)  [unwired: 1 out]
        n114 = String To Path(string=w406) -> (path=w401:path)
        n115 = case shown="\"d\", Default" w392 {
          tunnel: [w422 w423] -> w390
          frame "s" {
            w422 = u16 0 items=["Single", "Double"] ("sweep mode")
          }
          frame "d", Default {
            w423 = u16 1 items=["Single", "Double"] ("sweep mode")
          }
        }
        n116 = Fract/Exp String To Number(string=w391) -> (number=w373:dbl[])  [unwired: 3 in, 1 out]
        n117 = Index Array(array=w373, index #1=0 ("Index")) -> (element #1=w389:dbl, element #2=w388:dbl, element #3=w387:dbl)  [unwired: 2 in]
        n118 = Delete From Array(array=w373, length=3 ("Length"), index=0 ("Index")) -> (array with subset deleted=w372:dbl[])  [unwired: 1 out]
        n119 = Bundle By Name(cluster=w381, "Gate Start"=w389, "Gate Stop"=w388, "Gate Step (linear only)"=w387, "Gate Compliance"=w399, "Range mode"=w365, "Range"=w364) -> (w420:T3)
        n120 = Index Array(array=w372, index #1=0 ("Index")) -> (element #1=w384:dbl, element #2=w383:dbl, element #3=w382:dbl)  [unwired: 2 in]
        n121 = call <vilib>:"compatOverwrite.vi"("overwrite (F)"=TRUE) -> ("overwrite?"=w355:T7)
        n122 = Bundle By Name(cluster=w380, "Drain Start"=w384, "Drain Stop"=w383, "Drain Step"=w382, "Drain Compliance"=w400, "Range mode"=w363, "Range"=w366) -> (w419:T4)
        n123 = call <userlib>:"4155C Output.vi"("VISA resource name in"=w369, "Gate"=w420, "Drain"=w419, "Timings"=w398, "error in (no error)"=w368, "SMU4"=w357, "sweep mode"=w390, "Panel controls"=w421) -> ("VD"=w407:dbl[], "Outparams"=w360:T8, "VISA Resource Name out"=w396:refnum<visa-resource-name>, "IS"=w410:dbl[], "ID"=w409:dbl[], "IG"=w408:dbl[], "error out"=w397:errorcluster, "SMU4"=w356:dbl[])  [unwired: 12 in]
        n124 = Unbundle By Name(w360) -> ("V2 Step"=w361:dbl, "V2 Start"=w359:dbl, "Number of points"=w358:i32)
        n125 = Open/Create/Replace File(file path (use dialog)=w401, error in=w397, operation (0:open)=w355) -> (refnum out=w416:refnum<file>, error out=w417:errorcluster)  [unwired: 3 in, 1 out]
        n126 = call <userlib>:"4155C Make Big 2d array.vi"("1D Var1"=w407, "1d IS"=w410, "1d ID"=w409, "1d IG"=w408, "1d SMU4"=w356, "SMU4"=w357, "VAR2 START"=w359, "Number of VAR2 steps"=w358, "VAR2 STEP"=w361, "VAR1 Name"="Vd", "Decimal places in header"=i8 1, "VAR2 Name"="Vg") -> ("Header array"=w412:string[], "Data array"=w413:dbl[][])  [unwired: 14 in]
        n127 = call <userlib>:"4155C Write array to file.vi"("Byte Stream File Refnum"=w416, "Header"=w412, "Data Array"=w413, "error in (no error)"=w417) -> ("dup refnum"=w414:refnum<file>, "error out"=w415:errorcluster)  [unwired: 1 in]
        n128 = Close File(refnum=w414, error in=w415) -> (error out=w395:errorcluster)  [unwired: 1 out]
      }
      frame "output-fpp" {
        n129 = Number To Decimal String(number=w476) -> (decimal integer string=w477:string)  [unwired: 1 in]
        n130 = Bundle By Name(cluster=w452, "Emergency Stop"=w480) -> (w490:T6)
        n131 = Delete From Array(array=w467, index=0 ("Index")) -> (deleted portion=w465:string, array with subset deleted=w464:string[])  [unwired: 1 in]
        n132 = Concatenate Strings(w475, "-outputfpp-" ("Substring"), w477, ".txt" ("Substring")) -> (w479:string)
        n133 = VISA Write(VISA resource name=w443, write buffer=":PAGE:CHAN:MODE SWE;" ("write buffer (\"\")"), error in (no error)=w440) -> (VISA resource name out=w442:refnum<visa-resource-name>, error out=w441:errorcluster)  [unwired: 1 out]
        n134 = String To Path(string=w479) -> (path=w474:path)
        n135 = case shown="\"d\", Default" w465 {
          tunnel: [w491 w492] -> w463
          frame "s" {
            w491 = u16 0 items=["Single", "Double"] ("sweep mode")
          }
          frame "d", Default {
            w492 = u16 1 items=["Single", "Double"] ("sweep mode")
          }
        }
        n136 = Fract/Exp String To Number(string=w464) -> (number=w446:dbl[])  [unwired: 3 in, 1 out]
        n137 = Index Array(array=w446, index #1=0 ("Index")) -> (element #1=w462:dbl, element #2=w461:dbl, element #3=w460:dbl)  [unwired: 2 in]
        n138 = Delete From Array(array=w446, length=3 ("Length"), index=0 ("Index")) -> (array with subset deleted=w445:dbl[])  [unwired: 1 out]
        n139 = Bundle By Name(cluster=w454, "Gate Start"=w462, "Gate Stop"=w461, "Gate Step (linear only)"=w460, "Gate Compliance"=w472, "Range mode"=w438, "Range"=w437) -> (w489:T3)
        n140 = Index Array(array=w445, index #1=0 ("Index")) -> (element #1=w457:dbl, element #2=w456:dbl, element #3=w455:dbl)  [unwired: 2 in]
        n141 = call <vilib>:"compatOverwrite.vi"("overwrite (F)"=TRUE) -> ("overwrite?"=w425:T7)
        n142 = Bundle By Name(cluster=w453, "Drain Start"=w457, "Drain Stop"=w456, "Drain Step"=w455, "Drain Compliance"=w473, "Range mode"=w436, "Range"=w439) -> (w488:T4)
        n143 = call <userlib>:"4155C Output-FPP.vi"("VISA resource name in"=w442, "Gate"=w489, "Drain"=w488, "Timings"=w471, "error in (no error)"=w441, "sweep mode"=w463, "Panel controls"=w490) -> ("VD"=w430:dbl[], "Outparams"=w433:T8, "VISA Resource Name out"=w469:refnum<visa-resource-name>, "Vprobe2"=w429:dbl[], "ID"=w428:dbl[], "IG"=w427:dbl[], "Vprobe1"=w426:dbl[], "error out"=w470:errorcluster)  [unwired: 13 in]
        n144 = Unbundle By Name(w433) -> ("V2 Step"=w434:dbl, "V2 Start"=w432:dbl, "Number of points"=w431:i32)
        n145 = Open/Create/Replace File(file path (use dialog)=w474, error in=w470, operation (0:open)=w425) -> (refnum out=w485:refnum<file>, error out=w486:errorcluster)  [unwired: 3 in, 1 out]
        n146 = call <userlib>:"4155C Make Big 2d array FPP.vi"("1D Var1"=w430, "1d ID"=w428, "1d Vp2"=w429, "1d IG"=w427, "1d Vp1"=w426, "VAR2 START"=w432, "Number of VAR2 steps"=w431, "VAR2 STEP"=w434, "VAR1 Name"="Vd", "Decimal places in header"=i8 1, "VAR2 Name"="Vg") -> ("Header array"=w481:string[], "Data array"=w482:dbl[][])  [unwired: 15 in]
        n147 = call <userlib>:"4155C Write array to file.vi"("Byte Stream File Refnum"=w485, "Header"=w481, "Data Array"=w482, "error in (no error)"=w486) -> ("dup refnum"=w483:refnum<file>, "error out"=w484:errorcluster)  [unwired: 1 in]
        n148 = Close File(refnum=w483, error in=w484) -> (error out=w468:errorcluster)  [unwired: 1 out]
      }
      frame "itime" {
        n149 = Delete From Array(array=w505, index=0 ("Index")) -> (deleted portion=w506:string)  [unwired: 1 in, 1 out]
        n150 = case shown="\"l\"" w506 {
          tunnel: w504 -> [w510 w512 w515]
          tunnel: [w509 w511 w514] -> w497
          frame "s" {
            w508 = u32 0 items=["short  ", "medium  ", "long  "] ("integration time 2")
            n151 = Bundle By Name(cluster=w510, "integration time"=w508) -> (w509:T5)
          }
          frame "m", Default {
            w513 = u32 1 items=["short  ", "medium  ", "long  "] ("integration time 2")
            n152 = Bundle By Name(cluster=w512, "integration time"=w513) -> (w511:T5)
          }
          frame "l" {
            w516 = u32 2 items=["short  ", "medium  ", "long  "] ("integration time 2")
            n153 = Bundle By Name(cluster=w515, "integration time"=w516) -> (w514:T5)
          }
        }
      }
      frame "pulsed" {
        n154 = Delete From Array(array=w530, index=0 ("Index")) -> (deleted portion=w531:string, array with subset deleted=w518:string[])  [unwired: 1 in]
        n155 = case shown="\"on\", Default" w531 {
          tunnel: w529 -> [w541 w544]
          tunnel: [w540 w543] -> w522
          tunnel: w518 -> [w538 _]
          frame "on", Default {
            w539 = u16 1 items=["Continuous", "Pulsed"] ("sweep method")
            n156 = Fract/Exp String To Number(string=w538) -> (number=w536:dbl[])  [unwired: 3 in, 1 out]
            n157 = Index Array(array=w536, index #1=0 ("Index")) -> (element #1=w535:dbl, element #2=w534:dbl, element #3=w533:dbl)  [unwired: 2 in]
            n158 = Bundle By Name(cluster=w541, "sweep method"=w539, "Pulse period"=w535, "Base voltage"=w534, "Pulse width"=w533) -> (w540:T5)
          }
          frame "off" {
            w542 = u16 0 items=["Continuous", "Pulsed"] ("sweep method")
            n159 = Bundle By Name(cluster=w544, "sweep method"=w542) -> (w543:T5)
          }
        }
      }
      frame "gaterangemode" {
        n160 = Delete From Array(array=w556, index=0 ("Index")) -> (deleted portion=w557:string)  [unwired: 1 in, 1 out]
        n161 = case shown="\"f\"" w557 {
          tunnel: [w559 w560 w561] -> w546
          frame "a", Default {
            w559 = u16 0 items=["Auto", "Limited", "Fixed"] ("Gate Range\nmode 2")
          }
          frame "f" {
            w560 = u16 2 items=["Auto", "Limited", "Fixed"] ("Gate Range\nmode 2")
          }
          frame "l" {
            w561 = u16 1 items=["Auto", "Limited", "Fixed"] ("Gate Range\nmode 2")
          }
        }
      }
      frame "gaterange" {
        (unwired) u8 11 items=["10fA  ", "100fA  ", "1nA  ", "10nA", "100nA", "1uA", "10uA", "100uA", "1mA", "10mA", "100mA", "1A"] ("Gate Range 2")
        n162 = Delete From Array(array=w580, index=0 ("Index")) -> (deleted portion=w570:string)  [unwired: 1 in, 1 out]
        n163 = Scan Value(string=w570, format string="") -> (value=w568:dbl)  [unwired: 1 in, 1 out]
        n164 = Logarithm Base 10(1:w568) -> (0:w567:dbl)
        n165 = Round To Nearest(number=w567) -> (nearest integer value=w566:dbl)
        n166 = Add(x=w566, y=11.0) -> (x+y=w564:dbl)
        n167 = To Unsigned Byte Integer(number=w564) -> (unsigned 8bit integer=w563:u8)
      }
      frame "drainrange" {
        (unwired) u8 11 items=["10fA  ", "100fA  ", "1nA  ", "10nA", "100nA", "1uA", "10uA", "100uA", "1mA", "10mA", "100mA", "1A"] ("Gate Range 2")
        n168 = Delete From Array(array=w600, index=0 ("Index")) -> (deleted portion=w591:string)  [unwired: 1 in, 1 out]
        n169 = Scan Value(string=w591, format string="") -> (value=w589:dbl)  [unwired: 1 in, 1 out]
        n170 = Logarithm Base 10(1:w589) -> (0:w588:dbl)
        n171 = Round To Nearest(number=w588) -> (nearest integer value=w587:dbl)
        n172 = Add(x=w587, y=11.0) -> (x+y=w585:dbl)
        n173 = To Unsigned Byte Integer(number=w585) -> (unsigned 8bit integer=w584:u8)
      }
      frame "drainrangemode" {
        n174 = Delete From Array(array=w613, index=0 ("Index")) -> (deleted portion=w614:string)  [unwired: 1 in, 1 out]
        n175 = case shown="\"f\"" w614 {
          tunnel: [w616 w617 w618] -> w603
          frame "a", Default {
            w616 = u16 0 items=["Auto", "Limited", "Fixed"] ("Gate Range\nmode 2")
          }
          frame "f" {
            w617 = u16 2 items=["Auto", "Limited", "Fixed"] ("Gate Range\nmode 2")
          }
          frame "l" {
            w618 = u16 1 items=["Auto", "Limited", "Fixed"] ("Gate Range\nmode 2")
          }
        }
      }
      frame "Error", Default {
      }
      frame "logfile" {
        n176 = Number To Decimal String(number=w661) -> (decimal integer string=w665:string)  [unwired: 1 in]
        n177 = Concatenate Strings(w663, "logfile" ("Substring"), w665, ".txt" ("Substring")) -> (w660:string)
        n178 = String To Path(string=w660) -> (path=w633:path)
        n179 = Unbundle(w659) -> ("integration time"=w658:u32, "Short/Long integration time"=w657:dbl, "hold time (sec)"=w656:dbl, "delay time (sec)"=w655:dbl, "Step Time (0 disables)"=w654:dbl, "sweep method"=w653:u16, "Pulse period"=w652:dbl, "Base voltage"=w651:dbl, "Pulse width"=w650:dbl)
        n180 = Build Array(w658, w657, w656, w655, w654, w653, w652, w651, w650, w644, w645, w646, w647, w648, w649) -> (w637:dbl[])
        n181 = Insert Into Array(array=dbl[][] [] ("Input Array"), new element=w637) -> (w636:dbl[][])  [unwired: 2 in]
        n182 = call <vilib>:"compatOverwrite.vi"("overwrite (F)"=TRUE) -> ("overwrite?"=w631:T7)
        n183 = Open/Create/Replace File(file path (use dialog)=w633, error in=w635, operation (0:open)=w631) -> (refnum out=w641:refnum<file>, error out=w640:errorcluster)  [unwired: 3 in, 1 out]
        n184 = call <userlib>:"4155C Write array to file.vi"("Byte Stream File Refnum"=w641, "Header"=string[] ["Int Time", "Short/Long Itime", "Hold time", "Delay time", "Step time", "Sweep method", "Pulse period", "Base Voltage", "Pulse width", "Drain compliance", "Gate compliance", "Gate range mode", "Gate range", "S/D range mode", "S/D range"], "Data Array"=w636, "error in (no error)"=w640) -> ("dup refnum"=w643:refnum<file>, "error out"=w642:errorcluster)  [unwired: 1 in]
        n185 = Close File(refnum=w643, error in=w642) -> (error out=w634:errorcluster)  [unwired: 1 out]
      }
      frame "sample" {
        n186 = Number To Decimal String(number=w715) -> (decimal integer string=w714:string)  [unwired: 1 in]
        n187 = Fract/Exp String To Number(string=w711) -> (number=w671:dbl[])  [unwired: 3 in, 1 out]
        n188 = Concatenate Strings(w689, "-sample-" ("Substring"), w714, ".txt" ("Substring")) -> (w712:string)
        n189 = String To Path(string=w712) -> (path=w693:path)
        n190 = Index Array(array=w671, index=0 ("Index")) -> (element=w709:dbl)
        n191 = Index Array(array=w671, index=2 ("Index")) -> (element=w705:dbl)
        n192 = Index Array(array=w671, index=3 ("Index")) -> (element=w674:dbl)
        n193 = Index Array(array=w671, index=4 ("Index")) -> (element=w670:dbl)
        n194 = call <userlib>:"4155C Config Sampling Measurements.vi"("Sampling interval"=w670, "Sample time"=w674, "Display on/off"=TRUE, "Timings"=w680, "Num Points"=w705, "error in (no error)"=w717, "Drain Compliance"=w716, "Gate Compliance"=w690, "VISA session"=w718) -> ("error out"=w719:errorcluster, "dup VISA resource name"=w720:refnum<visa-resource-name>)  [unwired: 1 in]
        n195 = Index Array(array=w671, index=1 ("Index")) -> (element=w706:dbl)
        n196 = call <userlib>:"4155C Take Sample.vi"("Emergency Stop"=w686, "error in (no error)"=w719, "Vd"=w706, "Vg"=w709, "VISA resource name in"=w720) -> ("error out"=w684:errorcluster, "Id"=w722:dbl[], "Ig"=w695:dbl[], "VISA Resource Name out"=w682:refnum<visa-resource-name>, "Is"=w721:dbl[], "Time"=w699:dbl[])  [unwired: 1 in]
        n197 = Insert Into Array(array=dbl[][] [] ("Input Array"), new element=w699) -> (w698:dbl[][])  [unwired: 2 in]
        n198 = Insert Into Array(array=w698, new element=w695) -> (w697:dbl[][])  [unwired: 2 in]
        n199 = Insert Into Array(array=w697, new element=w722) -> (w696:dbl[][])  [unwired: 2 in]
        n200 = VISA Write(VISA resource name=w682, write buffer=":DISP ON" ("write buffer (\"\")"), error in (no error)=w684) -> (VISA resource name out=w681:refnum<visa-resource-name>, error out=w683:errorcluster)  [unwired: 1 out]
        n201 = Insert Into Array(array=w696, new element=w721) -> (w688:dbl[][])  [unwired: 2 in]
        n202 = Transpose 2D Array(2D array=w688) -> (transposed array=w687:dbl[][])
        n203 = call <vilib>:"compatOverwrite.vi"("overwrite (F)"=TRUE) -> ("overwrite?"=w668:T7)
        n204 = Open/Create/Replace File(file path (use dialog)=w693, error in=w683, operation (0:open)=w668) -> (refnum out=w702:refnum<file>, error out=w701:errorcluster)  [unwired: 3 in, 1 out]
        n205 = call <userlib>:"4155C Write array to file.vi"("Byte Stream File Refnum"=w702, "Header"=string[] ["Time /s", "Ig /A", "Id /A", "Is /A"], "Data Array"=w687, "error in (no error)"=w701) -> ("dup refnum"=w704:refnum<file>, "error out"=w703:errorcluster)  [unwired: 1 in]
        n206 = Close File(refnum=w704, error in=w703) -> (error out=w691:errorcluster)  [unwired: 1 out]
      }
      frame "samplei" {
        n207 = Number To Decimal String(number=w774) -> (decimal integer string=w773:string)  [unwired: 1 in]
        n208 = Fract/Exp String To Number(string=w770) -> (number=w736:dbl[])  [unwired: 3 in, 1 out]
        n209 = Concatenate Strings(w752, "-samplei-" ("Substring"), w773, ".txt" ("Substring")) -> (w771:string)
        n210 = String To Path(string=w771) -> (path=w755:path)
        n211 = Index Array(array=w736, index=4 ("Index")) -> (element=w730:dbl)
        n212 = Index Array(array=w736, index=3 ("Index")) -> (element=w731:dbl)
        n213 = Index Array(array=w736, index=1 ("Index")) -> (element=w733:dbl)
        n214 = Index Array(array=w736, index=0 ("Index")) -> (element=w734:dbl)
        n215 = Index Array(array=w736, index=2 ("Index")) -> (element=w732:dbl)
        n216 = call <userlib>:"4155C Config SamplingI Measurements.vi"("Sample time"=w732, "Display on/off"=TRUE, "Timings"=w744, "Num Points"=w733, "error in (no error)"=w776, "Sampling interval"=w731, "VISA session"=w777) -> ("error out"=w778:errorcluster, "dup VISA resource name"=w779:refnum<visa-resource-name>)  [unwired: 3 in]
        n217 = call <userlib>:"4155C Take SampleI.vi"("Emergency Stop"=w749, "error in (no error)"=w778, "Idg 2"=w734, "Vdg compliance 2"=w730, "VISA resource name in"=w779) -> ("error out"=w747:errorcluster, "Idg"=w781:dbl[], "Vdg"=w757:dbl[], "VISA Resource Name out"=w745:refnum<visa-resource-name>, "Is"=w780:dbl[], "Time"=w761:dbl[])  [unwired: 1 in]
        n218 = Insert Into Array(array=dbl[][] [] ("Input Array"), new element=w761) -> (w760:dbl[][])  [unwired: 2 in]
        n219 = Insert Into Array(array=w760, new element=w757) -> (w759:dbl[][])  [unwired: 2 in]
        n220 = Insert Into Array(array=w759, new element=w781) -> (w758:dbl[][])  [unwired: 2 in]
        n221 = VISA Write(VISA resource name=w745, write buffer=":DISP ON" ("write buffer (\"\")"), error in (no error)=w747) -> (VISA resource name out=w729:refnum<visa-resource-name>, error out=w746:errorcluster)  [unwired: 1 out]
        n222 = Insert Into Array(array=w758, new element=w780) -> (w751:dbl[][])  [unwired: 2 in]
        n223 = Transpose 2D Array(2D array=w751) -> (transposed array=w750:dbl[][])
        n224 = call <vilib>:"compatOverwrite.vi"("overwrite (F)"=TRUE) -> ("overwrite?"=w724:T7)
        n225 = Open/Create/Replace File(file path (use dialog)=w755, error in=w746, operation (0:open)=w724) -> (refnum out=w764:refnum<file>, error out=w763:errorcluster)  [unwired: 3 in, 1 out]
        n226 = call <userlib>:"4155C Write array to file.vi"("Byte Stream File Refnum"=w764, "Header"=string[] ["Time /s", "Vdg /V", "Idg /A", "Is /A"], "Data Array"=w750, "error in (no error)"=w763) -> ("dup refnum"=w766:refnum<file>, "error out"=w765:errorcluster)  [unwired: 1 in]
        n227 = Close File(refnum=w766, error in=w765) -> (error out=w727:errorcluster)  [unwired: 1 out]
        n228 = VISA Write(VISA resource name=w729, write buffer=";:PAGE:SCON:STAN OFF;:PAGE:CHAN:VSU2:DIS;" ("write buffer (\"\")"), error in (no error)=w727) -> (VISA resource name out=w725:refnum<visa-resource-name>, error out=w726:errorcluster)  [unwired: 1 out]
      }
      frame "#" {
        n229 = VISA Write(VISA resource name=w787, write buffer=":DISP ON" ("write buffer (\"\")"), error in (no error)=w786) -> (VISA resource name out=w785:refnum<visa-resource-name>, error out=w784:errorcluster)  [unwired: 1 out]
      }
      frame "stressV" {
        n230 = Number To Decimal String(number=w836) -> (decimal integer string=w835:string)  [unwired: 1 in]
        n231 = Fract/Exp String To Number(string=w832) -> (number=w804:dbl[])  [unwired: 3 in, 1 out]
        n232 = Concatenate Strings(w819, "-stressV-" ("Substring"), w835, ".txt" ("Substring")) -> (w833:string)
        n233 = String To Path(string=w833) -> (path=w823:path)
        n234 = Index Array(array=w804, index=3 ("Index")) -> (element=w801:dbl)
        n235 = Index Array(array=w804, index=1 ("Index")) -> (element=w799:dbl)
        n236 = Index Array(array=w804, index=0 ("Index")) -> (element=w798:dbl)
        n237 = Index Array(array=w804, index=4 ("Index")) -> (element=w803:dbl)
        n238 = Index Array(array=w804, index=2 ("Index")) -> (element=w800:dbl)
        n239 = call <userlib>:"4155C Config V Stress.vi"("VISA session"=w839, "ID compliance"=w801, "VD"=w799, "VG"=w798, "IG compliance"=w800, "error in (no error)"=w838, "Display on/off"=TRUE) -> ("dup VISA resource name"=w841:refnum<visa-resource-name>, "error out"=w840:errorcluster)
        n240 = call <userlib>:"4155C Apply Stress.vi"("error in (no error)"=w840, "Duration"=w803, "Emergency Stop"=w818, "VISA resource name in"=w841) -> ("error out"=w816:errorcluster, "VISA Resource Name out"=w814:refnum<visa-resource-name>)
        n241 = VISA Write(VISA resource name=w814, write buffer=":DISP ON" ("write buffer (\"\")"), error in (no error)=w816) -> (VISA resource name out=w813:refnum<visa-resource-name>, error out=w815:errorcluster)  [unwired: 1 out]
        n242 = call <vilib>:"compatOverwrite.vi"("overwrite (F)"=TRUE) -> ("overwrite?"=w797:T7)
        n243 = Open/Create/Replace File(file path (use dialog)=w823, error in=w815, operation (0:open)=w797) -> (refnum out=w826:refnum<file>, error out=w825:errorcluster)  [unwired: 3 in, 1 out]
        n244 = call <userlib>:"4155C Write array to file.vi"("Byte Stream File Refnum"=w826, "Header"=string[] ["V stress completed successfully", ""], "error in (no error)"=w825) -> ("dup refnum"=w828:refnum<file>, "error out"=w827:errorcluster)  [unwired: 2 in]
        n245 = Close File(refnum=w828, error in=w827) -> (error out=w821:errorcluster)  [unwired: 1 out]
      }
      frame "stressI" {
        n246 = Number To Decimal String(number=w878) -> (decimal integer string=w877:string)  [unwired: 1 in]
        n247 = Fract/Exp String To Number(string=w874) -> (number=w848:dbl[])  [unwired: 3 in, 1 out]
        n248 = Concatenate Strings(w861, "-stressI-" ("Substring"), w877, ".txt" ("Substring")) -> (w875:string)
        n249 = String To Path(string=w875) -> (path=w865:path)
        n250 = Index Array(array=w848, index=1 ("Index")) -> (element=w844:dbl)
        n251 = Index Array(array=w848, index=0 ("Index")) -> (element=w845:dbl)
        n252 = call <userlib>:"4155C Config I Stress.vi"("VISA session"=w881, "IDG"=w845, "VDG compliance"=w844, "error in (no error)"=w880, "Display on/off"=TRUE) -> ("dup VISA resource name"=w883:refnum<visa-resource-name>, "error out"=w882:errorcluster)
        n253 = Index Array(array=w848, index=2 ("Index")) -> (element=w846:dbl)
        n254 = call <userlib>:"4155C Apply Stress.vi"("error in (no error)"=w882, "Duration"=w846, "Emergency Stop"=w860, "VISA resource name in"=w883) -> ("error out"=w858:errorcluster, "VISA Resource Name out"=w856:refnum<visa-resource-name>)
        n255 = VISA Write(VISA resource name=w856, write buffer=":DISP ON" ("write buffer (\"\")"), error in (no error)=w858) -> (VISA resource name out=w855:refnum<visa-resource-name>, error out=w857:errorcluster)  [unwired: 1 out]
        n256 = call <vilib>:"compatOverwrite.vi"("overwrite (F)"=TRUE) -> ("overwrite?"=w843:T7)
        n257 = Open/Create/Replace File(file path (use dialog)=w865, error in=w857, operation (0:open)=w843) -> (refnum out=w868:refnum<file>, error out=w867:errorcluster)  [unwired: 3 in, 1 out]
        n258 = call <userlib>:"4155C Write array to file.vi"("Byte Stream File Refnum"=w868, "Header"=string[] ["I stress completed successfully", ""], "error in (no error)"=w867) -> ("dup refnum"=w870:refnum<file>, "error out"=w869:errorcluster)  [unwired: 2 in]
        n259 = Close File(refnum=w870, error in=w869) -> (error out=w863:errorcluster)  [unwired: 1 out]
      }
      frame "vsu2pulse" {
        n260 = Number To Decimal String(number=w918) -> (decimal integer string=w917:string)  [unwired: 1 in]
        n261 = Fract/Exp String To Number(string=w914) -> (number=w889:dbl[])  [unwired: 3 in, 1 out]
        n262 = Concatenate Strings(w902, "-vsu2-" ("Substring"), w917, ".txt" ("Substring")) -> (w915:string)
        n263 = String To Path(string=w915) -> (path=w906:path)
        n264 = Index Array(array=w889, index=1 ("Index")) -> (element=w888:dbl)
        n265 = Index Array(array=w889, index=0 ("Index")) -> (element=w886:dbl)
        n266 = call <userlib>:"4155C Config VSU2 Stress.vi"("error in (no error)"=w920, "VSU2"=w886, "Display on/off"=TRUE, "VISA session"=w921) -> ("error out"=w922:errorcluster, "dup VISA resource name"=w923:refnum<visa-resource-name>)
        n267 = call <userlib>:"4155C Apply Stress.vi"("error in (no error)"=w922, "Duration"=w888, "Emergency Stop"=w901, "VISA resource name in"=w923) -> ("error out"=w899:errorcluster, "VISA Resource Name out"=w897:refnum<visa-resource-name>)
        n268 = VISA Write(VISA resource name=w897, write buffer=":DISP ON" ("write buffer (\"\")"), error in (no error)=w899) -> (VISA resource name out=w896:refnum<visa-resource-name>, error out=w898:errorcluster)  [unwired: 1 out]
        n269 = call <vilib>:"compatOverwrite.vi"("overwrite (F)"=TRUE) -> ("overwrite?"=w885:T7)
        n270 = Open/Create/Replace File(file path (use dialog)=w906, error in=w898, operation (0:open)=w885) -> (refnum out=w909:refnum<file>, error out=w908:errorcluster)  [unwired: 3 in, 1 out]
        n271 = call <userlib>:"4155C Write array to file.vi"("Byte Stream File Refnum"=w909, "Header"=string[] ["VSU2 pulse completed successfully", ""], "error in (no error)"=w908) -> ("dup refnum"=w911:refnum<file>, "error out"=w910:errorcluster)  [unwired: 2 in]
        n272 = Close File(refnum=w911, error in=w910) -> (error out=w904:errorcluster)  [unwired: 1 out]
      }
      frame "sample-fpp" {
        w932 = string[] ["Time /s", "Id VgVd /A", "Ig VgVd /A", "Vp1 VgVd /V", "Vp2 VgVd /V"] ("Header")
        w936 = "%d" ("format string")
        n273 = Number To Decimal String(number=w986) -> (decimal integer string=w985:string)  [unwired: 1 in]
        n274 = Fract/Exp String To Number(string=w982) -> (number=w970:dbl[])  [unwired: 3 in, 1 out]
        n275 = Concatenate Strings(w976, "-samplefpp-" ("Substring"), w985, ".txt" ("Substring")) -> (w983:string)
        n276 = String To Path(string=w983) -> (path=w944:path)
        n277 = Index Array(array=w970, index=0 ("Index")) -> (element=w930:dbl)
        n278 = Index Array(array=w970, index=1 ("Index")) -> (element=w929:dbl)
        n279 = Index Array(array=w970, index=2 ("Index")) -> (element=w978:dbl)
        n280 = Index Array(array=w970, index=3 ("Index")) -> (element=w968:dbl)
        n281 = call <userlib>:"4155C Config Sampling Measurements FPP.vi"("VISA session"=w989, "Num Points"=w978, "Vg"=w930, "Display on/off"=TRUE, "Gate Compliance"=w977, "Drain Compliance"=w987, "Standby"="Standby", "error in (no error)"=w988, "Timings"=w975, "Vd"=w929, "Sample time"=w968) -> ("dup VISA resource name"=w946:refnum<visa-resource-name>, "error out"=w945:errorcluster)  [unwired: 3 in]
        n282 = Number To Decimal String(number=w930) -> (decimal integer string=w956:string)  [unwired: 1 in]
        n283 = call <userlib>:"4155C Take Sample FPP.vi"("VISA resource name in"=w946, "error in (no error)"=w945, "Emergency Stop"=w947) -> ("Time"=w951:dbl[], "Vp1"=w961:dbl[], "VISA Resource Name out"=w927:refnum<visa-resource-name>, "Ig"=w949:dbl[], "Id"=w950:dbl[], "Vp2"=w959:dbl[], "error out"=w948:errorcluster)  [unwired: 10 in]
        n284 = Insert Into Array(array=dbl[][] [] ("Input Array"), new element=w951) -> (w965:dbl[][])  [unwired: 2 in]
        n285 = Number To Decimal String(number=w929) -> (decimal integer string=w954:string)  [unwired: 1 in]
        n286 = Insert Into Array(array=w965, new element=w950) -> (w964:dbl[][])  [unwired: 2 in]
        n287 = Concatenate Strings("(Vg = " ("Substring"), w956, "V, Vd = " ("Substring"), w954, "V)" ("Substring")) -> (w952:string)
        n288 = Insert Into Array(array=w964, new element=w949) -> (w963:dbl[][])  [unwired: 2 in]
        n289 = Insert Into Array(array=w963, new element=w961) -> (w960:dbl[][])  [unwired: 2 in]
        n290 = Insert Into Array(array=w960, new element=w959) -> (w928:dbl[][])  [unwired: 2 in]
        n291 = call <vilib>:"compatOverwrite.vi"("overwrite (F)"=TRUE) -> ("overwrite?"=w925:T7)
        n292 = Open/Create/Replace File(file path (use dialog)=w944, error in=w948, operation (0:open)=w925) -> (refnum out=w941:refnum<file>, error out=w942:errorcluster)  [unwired: 3 in, 1 out]
        n293 = Array To Spreadsheet String(array=w932, 3:w936) -> (spreadsheet string=w938:string)  [unwired: 1 in]
        n294 = Transpose 2D Array(2D array=w928) -> (transposed array=w958:dbl[][])
        n295 = Search and Replace String(replace all?=TRUE ("replace all? (F)"), input string=w938, search string="VgVd", replace string=w952) -> (result string=w934:string)  [unwired: 4 in, 3 out]
        n296 = Spreadsheet String To Array(format string=w936, spreadsheet string=w934, array type (2D Dbl)=w932) -> (array=w933:string[])  [unwired: 1 in]
        n297 = call <userlib>:"4155C Write array to file.vi"("Byte Stream File Refnum"=w941, "Header"=w933, "Data Array"=w958, "error in (no error)"=w942) -> ("dup refnum"=w939:refnum<file>, "error out"=w940:errorcluster)  [unwired: 1 in]
        n298 = Close File(refnum=w939, error in=w940) -> (error out=w926:errorcluster)  [unwired: 1 out]
      }
      frame "resample-fpp" {
        w1000 = string[] ["Time /s", "Id VgVd /A", "Ig VgVd /A", "Vp1 VgVd /V", "Vp2 VgVd /V"] ("Header")
        w1004 = "%d" ("format string")
        n299 = Number To Decimal String(number=w1046) -> (decimal integer string=w1045:string)  [unwired: 1 in]
        n300 = Fract/Exp String To Number(string=w1042) -> (number=w993:dbl[])  [unwired: 3 in, 1 out]
        n301 = Concatenate Strings(w1038, "-resamplefpp-" ("Substring"), w1045, ".txt" ("Substring")) -> (w1043:string)
        n302 = String To Path(string=w1043) -> (path=w1012:path)
        n303 = Index Array(array=w993, index=0 ("Index")) -> (element=w999:dbl)
        n304 = Index Array(array=w993, index=1 ("Index")) -> (element=w998:dbl)
        n305 = Number To Decimal String(number=w999) -> (decimal integer string=w1022:string)  [unwired: 1 in]
        n306 = call <userlib>:"4155C Take Sample FPP.vi"("VISA resource name in"=w995, "error in (no error)"=w994, "Emergency Stop"=w1013) -> ("Time"=w1017:dbl[], "Vp1"=w1027:dbl[], "VISA Resource Name out"=w997:refnum<visa-resource-name>, "Ig"=w1015:dbl[], "Id"=w1016:dbl[], "Vp2"=w1025:dbl[], "error out"=w1014:errorcluster)  [unwired: 10 in]
        n307 = Insert Into Array(array=dbl[][] [] ("Input Array"), new element=w1017) -> (w1031:dbl[][])  [unwired: 2 in]
        n308 = Number To Decimal String(number=w998) -> (decimal integer string=w1020:string)  [unwired: 1 in]
        n309 = Insert Into Array(array=w1031, new element=w1016) -> (w1030:dbl[][])  [unwired: 2 in]
        n310 = Concatenate Strings("(Vg = " ("Substring"), w1022, "V, Vd = " ("Substring"), w1020, "V)" ("Substring")) -> (w1018:string)
        n311 = Insert Into Array(array=w1030, new element=w1015) -> (w1029:dbl[][])  [unwired: 2 in]
        n312 = Insert Into Array(array=w1029, new element=w1027) -> (w1026:dbl[][])  [unwired: 2 in]
        n313 = Insert Into Array(array=w1026, new element=w1025) -> (w992:dbl[][])  [unwired: 2 in]
        n314 = call <vilib>:"compatOverwrite.vi"("overwrite (F)"=TRUE) -> ("overwrite?"=w991:T7)
        n315 = Open/Create/Replace File(file path (use dialog)=w1012, error in=w1014, operation (0:open)=w991) -> (refnum out=w1009:refnum<file>, error out=w1010:errorcluster)  [unwired: 3 in, 1 out]
        n316 = Array To Spreadsheet String(array=w1000, 3:w1004) -> (spreadsheet string=w1006:string)  [unwired: 1 in]
        n317 = Transpose 2D Array(2D array=w992) -> (transposed array=w1024:dbl[][])
        n318 = Search and Replace String(replace all?=TRUE ("replace all? (F)"), input string=w1006, search string="VgVd", replace string=w1018) -> (result string=w1002:string)  [unwired: 4 in, 3 out]
        n319 = Spreadsheet String To Array(format string=w1004, spreadsheet string=w1002, array type (2D Dbl)=w1000) -> (array=w1001:string[])  [unwired: 1 in]
        n320 = call <userlib>:"4155C Write array to file.vi"("Byte Stream File Refnum"=w1009, "Header"=w1001, "Data Array"=w1024, "error in (no error)"=w1010) -> ("dup refnum"=w1007:refnum<file>, "error out"=w1008:errorcluster)  [unwired: 1 in]
        n321 = Close File(refnum=w1007, error in=w1008) -> (error out=w996:errorcluster)  [unwired: 1 out]
      }
    }
    n322 = local write "Lines left to run:"(w41) -> ()
    n323 = Empty String/Path?(string/path=w41) -> (empty?=w77:bool)
    n324 = Not(x=w77) -> (.not. x?=w76:bool)
  }
